vi "R2_Control.vi"() -> ()   [LabVIEW 2016]
uses:
  R2 Reactor Status v1.ctl
  R2 SBR Mode Control.ctl
  R2 pH Manual Control.ctl
  R2 Pump Manual Control.ctl
  R2 DO Manual Control.ctl
  R2Variables.lvlib
panel:
  in  "High DO Manual Control":cluster{"Air Valve":bool, "N2 Valve":bool}
  in  "High DO Control":T1={"DO set point (mg/L)"=2.0, "N2 Gain"=15.0, "Air Gain"=3.0, "DO Tolerance (mg/L)"=0.05, "Air Short Reaction Time (s)"=15.0, "Long Reaction Time (s)"=30.0, "N2 Short Reaction Time (s) 2"=10.0}
  out "Elapsed Time":dbl
  in  "Main DO Control":T1={"DO set point (mg/L)"=2.0, "N2 Gain"=15.0, "Air Gain"=5.0, "DO Tolerance (mg/L)"=0.05, "Air Short Reaction Time (s)"=15.0, "Long Reaction Time (s)"=30.0, "N2 Short Reaction Time (s) 2"=10.0}
  out "pH and DO":cluster{"pH":dbl, "DO (mg/L)":dbl}(graph)
  out "DO Intercept":dbl
  out "DO Slope":dbl
  out "pH Intercept":dbl
  out "pH Slope":dbl
  in  "DO Control":T2
  in  "Reactor 2 Pumps Manual Control":T3
  in  "pH Control":T4
  in  "pH Control":T5={" pH Set Point"=7.5, " pH Tolerance"=0.1, "Reaction Time (s)"=15.0, "Pump On Time (s)"=3.0}
  in  "SBR Timing":T6={"Anaerobic Feed"=60.0, "Aerobic"=180.0, "Settle 1"=3.0, "Floc Decant 1"=1.0, "Mix 2"=1.0, "Idle"=13.0, "Aerobic no DO control "=2.0, "Settle 2 (min)"=2.0, "Floc Decant 2"=1.0, "Mix 3"=1.0, "Settle 3"=1.0, "Floc Decant 3"=1.0, "Water Fill + Floc Return"=2.0, "High DO"=60.0, "N2 Purge"=5.0, "Effluent"=2.0}
  out "N2 and Air Flow":cluster{"N2 Flow":dbl, "Air Flow":dbl}(graph)
  out "Reactor 2 Status":T7 {"Compressed Air" format="%#.0g"; "Release Flow" format="%#.0g"; "DO Amp (A)" format="%#.4g"; "pH Amp (A)" format="%#.4g"; "DO (mg/L)" format="%#.2g"; "pH" format="%#.2g"}
  in  "Pumps Manual Control":bool
  in  "DO Manual Control":bool
  in  "pH Manual Control":bool
  in  "DO Calibrate":bool
  in  "pH Calibrate":bool
  # "On: Manual Mode\nOff: SBR Mode"
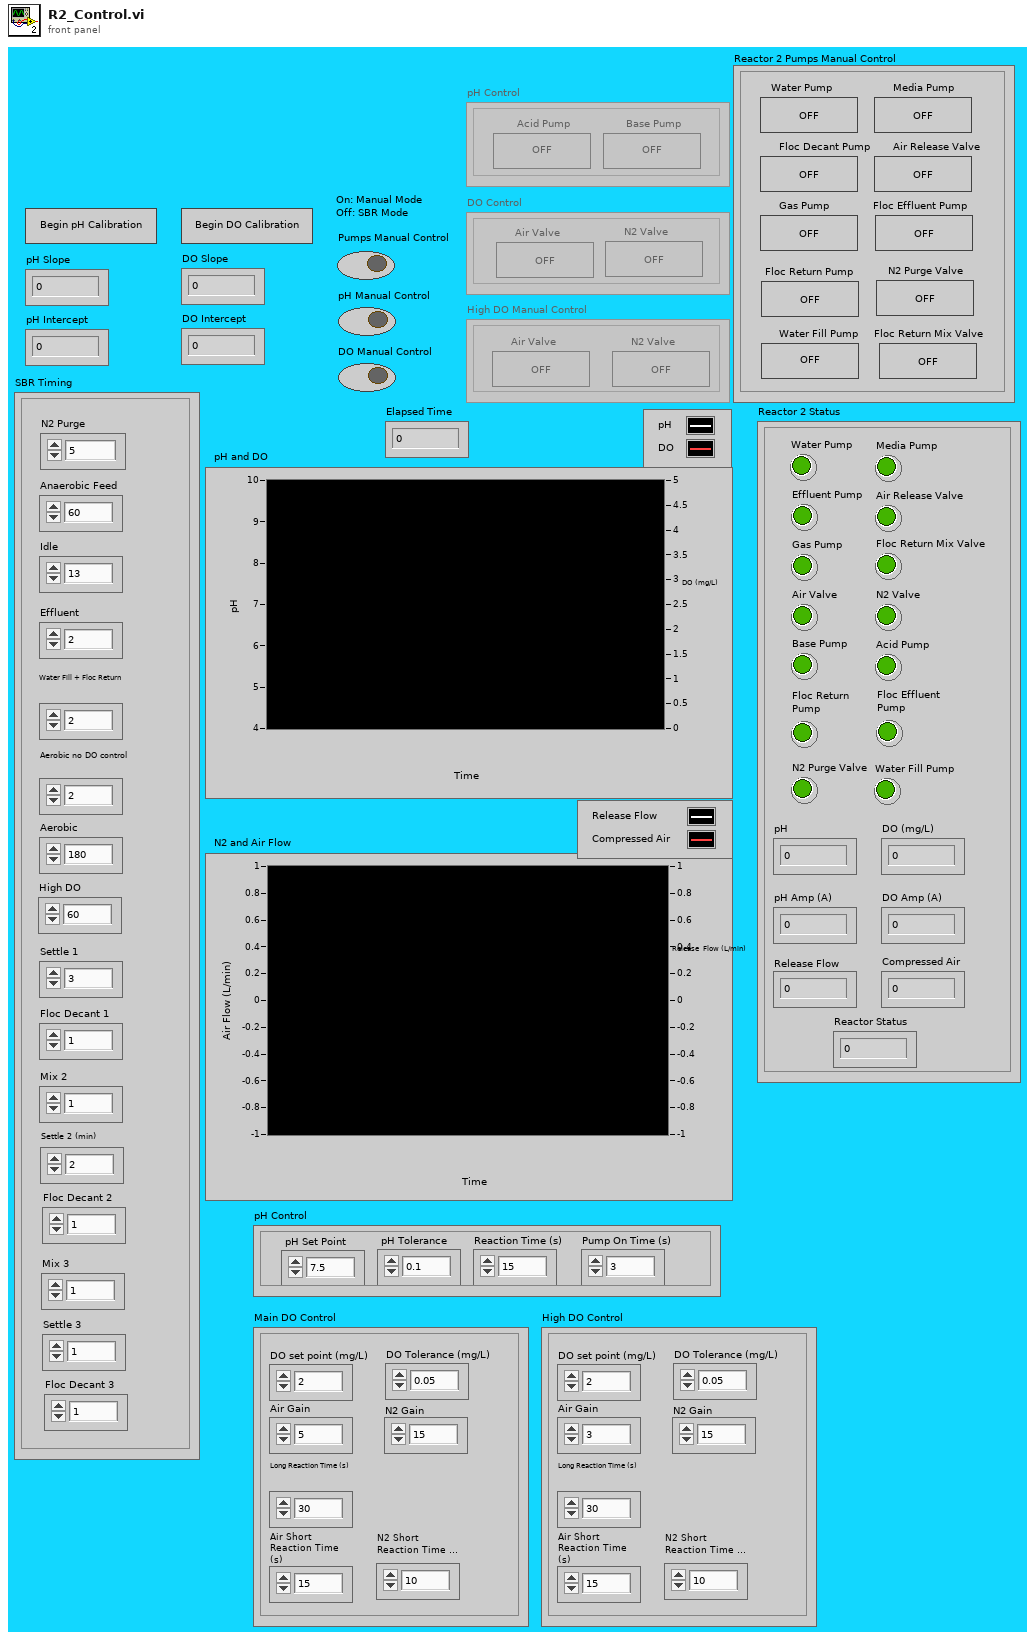
[diagram p1: front panel]
types:
  T1 = cluster{"DO set point (mg/L)":dbl, "N2 Gain":dbl, "Air Gain":dbl, "DO Tolerance (mg/L)":dbl, "Air Short Reaction Time (s)":dbl, "Long Reaction Time (s)":dbl, "N2 Short Reaction Time (s) 2":dbl}
  T2 = typedef "R2Variables.lvlib/R2 DO Manual Control.ctl" = cluster{"Air Valve":bool, "N2 Valve":bool}
  T3 = typedef "R2Variables.lvlib/R2 Pump Manual Control.ctl" = cluster{"Water Fill Pump":bool, "Floc Decant Pump":bool, "Media Pump":bool, "Gas Pump":bool, "Air Release Valve":bool, "Floc Effluent Pump":bool, "Floc Return Pump":bool, "N2 Purge Valve":bool, "Water Pump":bool, "Floc Return Mix Valve":bool}
  T4 = typedef "R2Variables.lvlib/R2 pH Manual Control.ctl" = cluster{"Acid Pump":bool, "Base Pump":bool}
  T5 = cluster{" pH Set Point":dbl, " pH Tolerance":dbl, "Reaction Time (s)":dbl, "Pump On Time (s)":dbl}
  T6 = typedef "R2Variables.lvlib/R2 SBR Mode Control.ctl" = cluster{"Anaerobic Feed":dbl, "Aerobic":dbl, "Settle 1":dbl, "Floc Decant 1":dbl, "Mix 2":dbl, "Idle":dbl, "Aerobic no DO control ":dbl, "Settle 2 (min)":dbl, "Floc Decant 2":dbl, "Mix 3":dbl, "Settle 3":dbl, "Floc Decant 3":dbl, "Water Fill + Floc Return":dbl, "High DO":dbl, "N2 Purge":dbl, "Effluent":dbl}
  T7 = typedef "R2Variables.lvlib/R2 Reactor Status v1.ctl" = cluster{"Water Fill Pump":bool, "Media Pump":bool, "Effluent Pump":bool, "Base Pump":bool, "Gas Pump":bool, "Acid Pump":bool, "Air Release Valve":bool, "N2 Valve":bool, "pH":dbl, "DO (mg/L)":dbl, "pH Amp (A)":dbl, "DO Amp (A)":dbl, "Release Flow":dbl, "Compressed Air":dbl, "Reactor Status":sgl, "Air Valve":bool, "Floc Return \nPump":bool, "Floc Effluent\nPump ":bool, "N2 Purge Valve":bool, "Water Pump":bool, "Floc Return Mix Valve":bool}
  T8 = enum8{"Enabled", "Disabled", "Disabled and Grayed Out"}
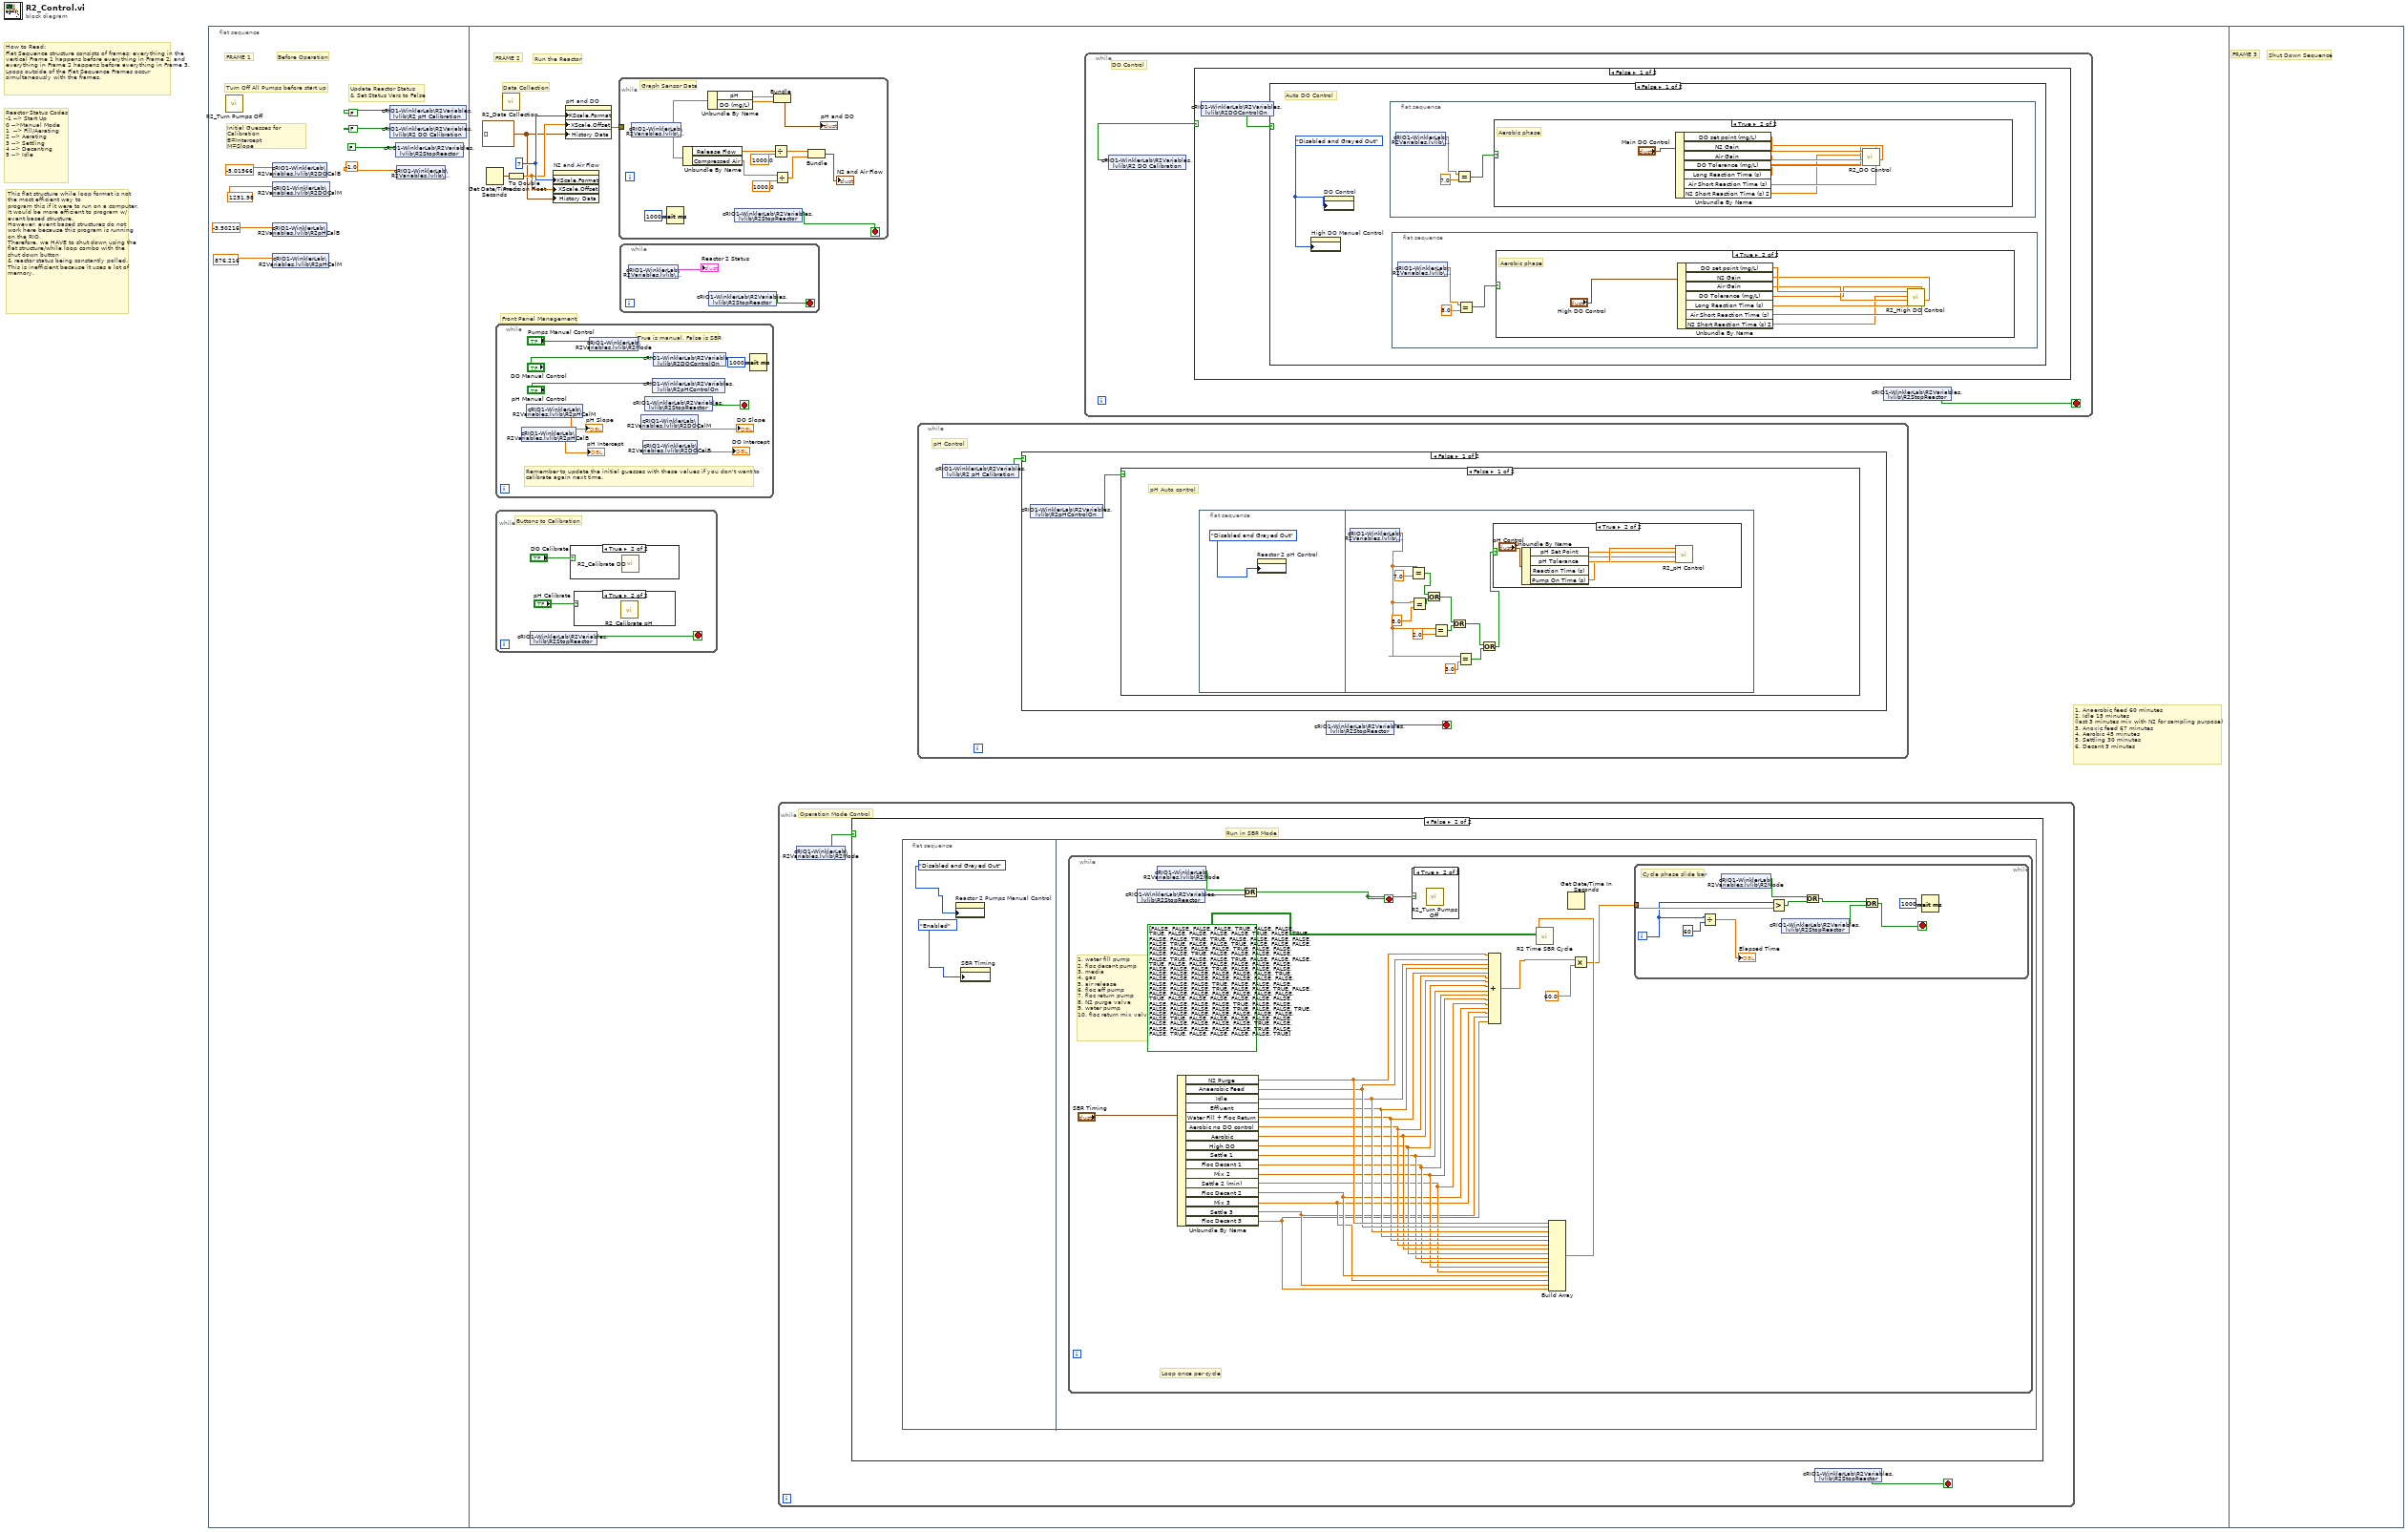
[diagram p0: block diagram]
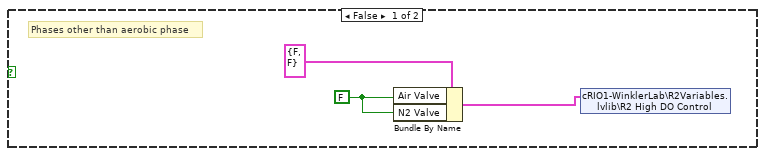
[diagram p2: hidden frame]
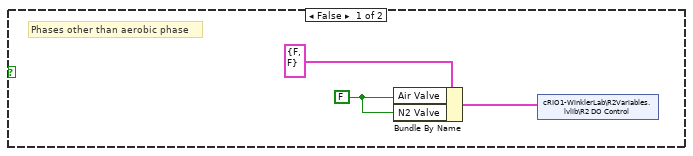
[diagram p3: hidden frame]
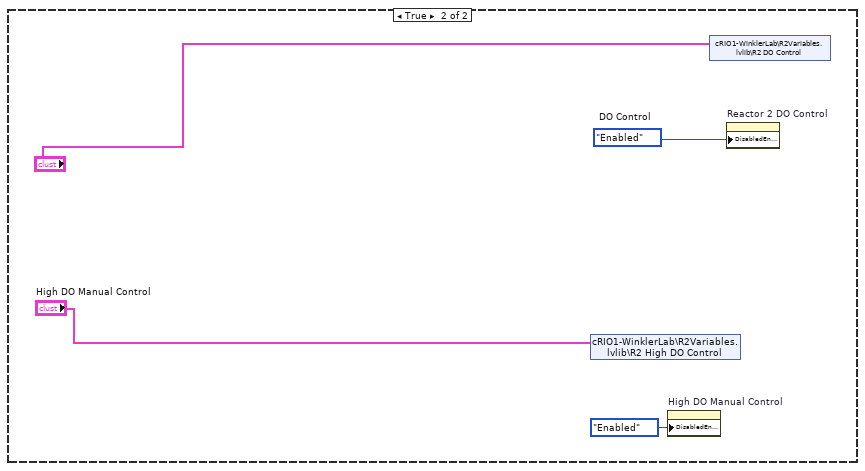
[diagram p4: hidden frame]
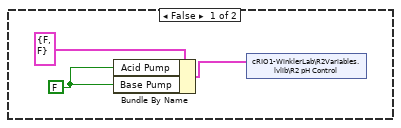
[diagram p8: hidden frame]
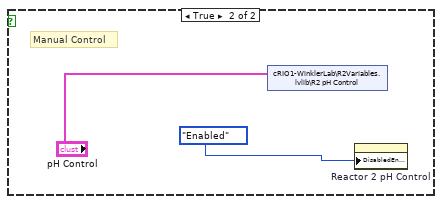
[diagram p9: hidden frame]
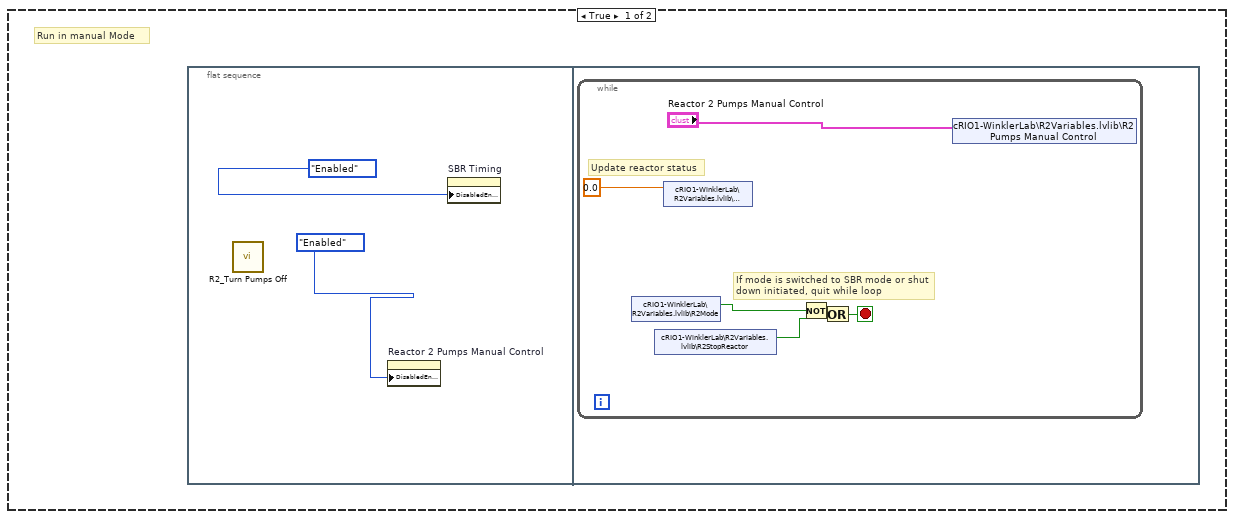
[diagram p11: hidden frame]
diagram:
  # "Reactor Status Codes\n-1 --> Start Up\n0 -->Manual Mode\n1  --> Fill/Aerating\n2 --> Aerating\n3 --> Settling\n4 --> Decanting\n5 --> Idle"
  # "How to Read:\nFlat Sequence structure consists of frames; everything in the vertical Frame 1 happens before everything in Frame 2, and everything in Frame 2 happens before everything in Frame 3.\nLoops outside of the Flat Sequence Frames occur simultaneously with the frames."
  # "This flat structure while loop format is not the most efficient way to \nprogram this if it were to run on a computer.\nIt would be more efficient to program w/ event based structure.\nHowever, event based structures do not work here because this program is running on the RIO.\nTherefore, we HAVE to shut down using the flat structure/while loop combo with the shut down button \n& reactor status being constantly polled.\nThis is inefficient because it uses a lot of memory."
  n1 = flat-sequence {
    frame #0 {
      # "Initial Guesses for Calibration\nB=Intercept\nM=Slope"
      # "Update Reactor Status \n& Set Status Vars to False"
      # "Turn Off All Pumps before start up"
      # "FRAME 1"
      # "Before Operation"
      n2 = call "R2_Turn Pumps Off.vi"() -> ()  [unwired: 12 in]
      n3 = shared-variable "cRIO1-WinklerLab\\R2Variables.lvlib\\R2DOCalB"(-5.01566 ("R1DOxCalB")) -> ()  [unwired: 1 in, 1 out]
      n4 = shared-variable "cRIO1-WinklerLab\\R2Variables.lvlib\\R2DOCalM"(1251.98 ("R1DOxCalM")) -> ()  [unwired: 1 in, 1 out]
      n5 = shared-variable "cRIO1-WinklerLab\\R2Variables.lvlib\\R2pHCalB"(-3.50216 ("R1pHCalB")) -> ()  [unwired: 1 in, 1 out]
      n6 = shared-variable "cRIO1-WinklerLab\\R2Variables.lvlib\\R2pHCalM"(876.216 ("R1pHCalM")) -> ()  [unwired: 1 in, 1 out]
      n7 = shared-variable "cRIO1-WinklerLab\\R2Variables.lvlib\\R2 pH Calibration"(FALSE ("pH Calibration")) -> ()  [unwired: 1 in, 1 out]
      n8 = shared-variable "cRIO1-WinklerLab\\R2Variables.lvlib\\R2 DO Calibration"(FALSE ("DO Calibration")) -> ()  [unwired: 1 in, 1 out]
      n9 = shared-variable "cRIO1-WinklerLab\\R2Variables.lvlib\\R2StopReactor"(FALSE ("R1Stop Reactor")) -> ()  [unwired: 1 in, 1 out]
      n10 = shared-variable "cRIO1-WinklerLab\\R2Variables.lvlib\\R2Phase"(-1.0) -> ()  [unwired: 1 in, 1 out]
    }
    frame #1 {
      w9 = cluster{"pH":dbl, "DO (mg/L)":dbl}[] [] ("History Data")
      w11 = u8 7 ("X Scale.Display Format:Format")
      # "1. Anaerobic feed 60 minutes\n2. Idle 15 minutes \n(last 3 minutes mix with N2 for sampling purpose)\n3. Anoxic feed 67 minutes\n4. Aerobic 45 minutes\n5. Settling 30 minutes\n6. Decant 5 minutes"
      # "Front Panel Management"
      # "Data Collection"
      # "FRAME 2"
      # "Run the Reactor"
      n11 = Get Date/Time In Seconds() -> (seconds since 1Jan1904=w13:timestamp)
      n12 = while {
        stop <- w98 stop-if-true
        # "Remember to update the initial guesses with these values if you don't want to calibrate again next time."
        # "True is manual, False is SBR"
        n13 = shared-variable "cRIO1-WinklerLab\\R2Variables.lvlib\\R2pHCalB"() -> (→"pH Intercept":dbl)  [unwired: 1 in, 1 out]
        n14 = shared-variable "cRIO1-WinklerLab\\R2Variables.lvlib\\R2pHCalM"() -> (→"pH Slope":dbl)  [unwired: 1 in, 1 out]
        n15 = shared-variable "cRIO1-WinklerLab\\R2Variables.lvlib\\R2Mode"("Pumps Manual Control") -> ()  [unwired: 1 in, 1 out]
        n16 = shared-variable "cRIO1-WinklerLab\\R2Variables.lvlib\\R2DOCalM"() -> (→"DO Slope":dbl)  [unwired: 1 in, 1 out]
        n17 = shared-variable "cRIO1-WinklerLab\\R2Variables.lvlib\\R2DOCalB"() -> (→"DO Intercept":dbl)  [unwired: 1 in, 1 out]
        n18 = shared-variable "cRIO1-WinklerLab\\R2Variables.lvlib\\R2StopReactor"() -> (w98:bool)  [unwired: 1 in, 1 out]
        n19 = shared-variable "cRIO1-WinklerLab\\R2Variables.lvlib\\R2pHControlOn"("pH Manual Control") -> ()  [unwired: 1 in, 1 out]
        n20 = shared-variable "cRIO1-WinklerLab\\R2Variables.lvlib\\R2DOControlOn"("DO Manual Control") -> ()  [unwired: 1 in, 1 out]
        n21 = Wait (ms)(milliseconds to wait=u32 1000) -> ()  [unwired: 1 out]
      }
      n22 = while {
        stop <- w65 stop-if-true
        # "Buttons to Calibration"
        n23 = shared-variable "cRIO1-WinklerLab\\R2Variables.lvlib\\R2StopReactor"() -> (w65:bool)  [unwired: 1 in, 1 out]
        n24 = case shown="True" "DO Calibrate" {
          frame False {
          }
          frame True {
            n25 = call "R2_Calibrate DO.vi"() -> ()  [unwired: 12 in]
          }
        }
        n26 = case shown="True" "pH Calibrate" {
          frame False {
          }
          frame True {
            n27 = call "R2_Calibrate pH.vi"() -> ()  [unwired: 12 in]
          }
        }
      }
      n28 = call "R2_Data Collection.vi"() -> ()  [unwired: 12 in]
      n29 = To Double Precision Float(number=w13) -> (double precision float=w10:dbl)
      n30 = property on="N2 and Air Flow" class="WFChart (strict)"("XScale.Format"=w11, "XScale.Offset"=w10, "History Data"=w9) -> ()  [unwired: 2 in, 2 out]
      n31 = property on="pH and DO" class="WFChart (strict)"("XScale.Format"=w11, "XScale.Offset"=w10, "History Data"=w9) -> (error out=w12:errorcluster)  [unwired: 2 in, 1 out]
      n32 = while {
        tunnel: w12 -> [_]
        stop <- w24 stop-if-true
        # "Graph Sensor Data"
        n33 = shared-variable "cRIO1-WinklerLab\\R2Variables.lvlib\\R2Status"() -> (w25:T7)  [unwired: 1 in, 1 out]
        n34 = Wait (ms)(milliseconds to wait=u32 1000) -> ()  [unwired: 1 out]
        n35 = Unbundle By Name(w25) -> ("Release Flow"=w21:dbl, "Compressed Air"=w18:dbl)
        n36 = Unbundle By Name(w25) -> ("pH"=w26:dbl, "DO (mg/L)"=w27:dbl)
        n37 = shared-variable "cRIO1-WinklerLab\\R2Variables.lvlib\\R2StopReactor"() -> (w24:bool)  [unwired: 1 in, 1 out]
        n38 = Divide(x=w21, y=1000.0) -> (x/y=w17:dbl)
        n39 = Bundle("pH"=w26, "DO (mg/L)"=w27) -> (→"pH and DO":cluster{"pH":dbl, "DO (mg/L)":dbl})  [unwired: 1 in]
        n40 = Divide(x=w18, y=1000.0) -> (x/y=w16:dbl)
        n41 = Bundle(w17, w16) -> (→"N2 and Air Flow":cluster{dbl, dbl})  [unwired: 1 in]
      }
      n42 = while {
        stop <- w14 stop-if-true
        n43 = shared-variable "cRIO1-WinklerLab\\R2Variables.lvlib\\R2Status"() -> (→"Reactor 2 Status":T7)  [unwired: 1 in, 1 out]
        n44 = shared-variable "cRIO1-WinklerLab\\R2Variables.lvlib\\R2StopReactor"() -> (w14:bool)  [unwired: 1 in, 1 out]
      }
      n45 = while {
        stop <- w104 stop-if-true
        # "Operation Mode Control"
        n46 = shared-variable "cRIO1-WinklerLab\\R2Variables.lvlib\\R2Mode"() -> (w103:bool)  [unwired: 1 in, 1 out]
        n47 = case shown="False" w103 {
          frame True {
            # "Run in manual Mode"
            n48 = flat-sequence {
              frame #0 {
                n49 = call "R2_Turn Pumps Off.vi"() -> ()  [unwired: 12 in]
                n50 = property on="Reactor 2 Pumps Manual Control" class="Clust (strict)"("DisabledEnum"=T8."Enabled" ("Disabled")) -> ()  [unwired: 2 in, 2 out]
                n51 = property on="SBR Timing" class="Clust (strict)"("DisabledEnum"=T8."Enabled" ("Disabled")) -> ()  [unwired: 2 in, 2 out]
              }
              frame #1 {
                n52 = while {
                  stop <- w111 stop-if-true
                  # "If mode is switched to SBR mode or shut \ndown initiated, quit while loop"
                  # "Update reactor status"
                  n53 = shared-variable "cRIO1-WinklerLab\\R2Variables.lvlib\\R2Mode"() -> (w109:bool)  [unwired: 1 in, 1 out]
                  n54 = shared-variable "cRIO1-WinklerLab\\R2Variables.lvlib\\R2StopReactor"() -> (w108:bool)  [unwired: 1 in, 1 out]
                  n55 = shared-variable "cRIO1-WinklerLab\\R2Variables.lvlib\\R2Phase"(0.0 ("Reactor Status")) -> ()  [unwired: 1 in, 1 out]
                  n56 = Not(x=w109) -> (.not. x?=w112:bool)
                  n57 = Or(x=w112, y=w108) -> (x .or. y?=w111:bool)
                  n58 = shared-variable "cRIO1-WinklerLab\\R2Variables.lvlib\\R2 Pumps Manual Control"("Reactor 2 Pumps Manual Control") -> ()  [unwired: 1 in, 1 out]
                }
              }
            }
          }
          frame False {
            # "Run in SBR Mode"
            n59 = flat-sequence {
              frame #0 {
                n60 = property on="Reactor 2 Pumps Manual Control" class="Clust (strict)"("DisabledEnum"=T8."Disabled and Grayed Out" ("Disabled")) -> ()  [unwired: 2 in, 2 out]
                n61 = property on="SBR Timing" class="Clust (strict)"("DisabledEnum"=T8."Enabled" ("Disabled")) -> ()  [unwired: 2 in, 2 out]
              }
              frame #1 {
                n62 = while {
                  stop <- w139 stop-if-true
                  # "1. water fill pump \n2. floc decant pump\n3. media \n4. gas \n5. air release\n6. floc eff pump\n7. floc return pump\n8. N2 purge valve\n9. water pump\n10. floc return mix valve"
                  # "Loop once per cycle"
                  n63 = shared-variable "cRIO1-WinklerLab\\R2Variables.lvlib\\R2StopReactor"() -> (w137:bool)  [unwired: 1 in, 1 out]
                  n64 = shared-variable "cRIO1-WinklerLab\\R2Variables.lvlib\\R2Mode"() -> (w138:bool)  [unwired: 1 in, 1 out]
                  n65 = Unbundle By Name("SBR Timing") -> ("N2 Purge"=w130:dbl, "Anaerobic Feed"=w129:dbl, "Idle"=w128:dbl, "Effluent"=w127:dbl, "Water Fill + Floc Return"=w126:dbl, "Aerobic no DO control"=w125:dbl, "Aerobic"=w124:dbl, "High DO"=w123:dbl, "Settle 1"=w122:dbl, "Floc Decant 1"=w121:dbl, "Mix 2"=w120:dbl, "Settle 2 (min)"=w119:dbl, "Floc Decant 2"=w118:dbl, "Mix 3"=w117:dbl, "Settle 3"=w116:dbl, "Floc Decant 3"=w115:dbl)
                  n66 = Or(x=w138, y=w137) -> (x .or. y?=w139:bool)
                  n67 = case shown="True" w139 {
                    frame False {
                    }
                    frame True {
                      n68 = call "R2_Turn Pumps Off.vi"() -> ()  [unwired: 12 in]
                    }
                  }
                  n69 = Compound Arithmetic op=ADD(w130, w129, w128, w127, w126, w125, w124, w123, w122, w121, w120, w119, w118, w117, w116, w115) -> (w132:dbl)
                  n70 = Build Array(w130, w129, w128, w127, w126, w125, w124, w123, w122, w121, w120, w119, w118, w117, w116, w115) -> (w135:dbl[])
                  n71 = call "R2 Time SBR Cycle.vi"("Pump Status Array"=bool[][] [[FALSE, FALSE, FALSE, FALSE, TRUE, FALSE, FALSE, TRUE, FALSE, FALSE], [FALSE, FALSE, TRUE, FALSE, TRUE, FALSE, FALSE, TRUE, TRUE, FALSE], [FALSE, FALSE, FALSE, FALSE, TRUE, FALSE, FALSE, TRUE, FALSE, FALSE], [FALSE, FALSE, FALSE, FALSE, FALSE, TRUE, FALSE, FALSE, FALSE, FALSE], [TRUE, FALSE, FALSE, FALSE, FALSE, FALSE, TRUE, FALSE, FALSE, TRUE], [FALSE, FALSE, FALSE, TRUE, FALSE, FALSE, FALSE, FALSE, FALSE, FALSE], [FALSE, FALSE, FALSE, TRUE, FALSE, FALSE, FALSE, FALSE, FALSE, FALSE], [FALSE, FALSE, FALSE, TRUE, FALSE, FALSE, FALSE, FALSE, FALSE, FALSE], [FALSE, FALSE, FALSE, FALSE, TRUE, FALSE, FALSE, FALSE, FALSE, FALSE], [FALSE, TRUE, FALSE, FALSE, TRUE, FALSE, FALSE, FALSE, FALSE, FALSE], [FALSE, FALSE, FALSE, TRUE, FALSE, FALSE, FALSE, FALSE, FALSE, FALSE], [FALSE, FALSE, FALSE, FALSE, TRUE, FALSE, FALSE, FALSE, FALSE, FALSE], [FALSE, TRUE, FALSE, FALSE, TRUE, FALSE, FALSE, FALSE, FALSE, FALSE], [FALSE, FALSE, FALSE, TRUE, FALSE, FALSE, FALSE, FALSE, FALSE, FALSE], [FALSE, FALSE, FALSE, FALSE, TRUE, FALSE, FALSE, FALSE, FALSE, FALSE], [FALSE, TRUE, FALSE, FALSE, TRUE, FALSE, FALSE, FALSE, FALSE, TRUE]], "Array"=w135) -> ()  [unwired: 10 in]
                  n72 = Get Date/Time In Seconds() -> ()  [unwired: 1 out]
                  n73 = Multiply(x=w132, y=60.0) -> (x*y=w133:dbl)
                  n74 = while {
                    tunnel: w133 -> [w148]
                    i -> [w141]
                    stop <- w142 stop-if-true
                    # "Cycle phase slide bar"
                    n75 = Divide(x=w141, y=60) -> (x/y=→"Elapsed Time":dbl)
                    n76 = shared-variable "cRIO1-WinklerLab\\R2Variables.lvlib\\R2Mode"() -> (w145:bool)  [unwired: 1 in, 1 out]
                    n77 = Greater?(x=w141, y=w148) -> (0:w146:bool)
                    n78 = shared-variable "cRIO1-WinklerLab\\R2Variables.lvlib\\R2StopReactor"() -> (w143:bool)  [unwired: 1 in, 1 out]
                    n79 = Or(x=w145, y=w146) -> (x .or. y?=w144:bool)
                    n80 = Or(x=w144, y=w143) -> (x .or. y?=w142:bool)
                    n81 = Wait (ms)(milliseconds to wait=u32 1000) -> ()  [unwired: 1 out]
                  }
                }
              }
            }
          }
        }
        n82 = shared-variable "cRIO1-WinklerLab\\R2Variables.lvlib\\R2StopReactor"() -> (w104:bool)  [unwired: 1 in, 1 out]
      }
      n83 = while {
        stop <- w69 stop-if-true
        # "pH Control"
        n84 = shared-variable "cRIO1-WinklerLab\\R2Variables.lvlib\\R2 pH Calibration"() -> (w68:bool)  [unwired: 1 in, 1 out]
        n85 = case shown="False" w68 {
          frame False {
            n86 = shared-variable "cRIO1-WinklerLab\\R2Variables.lvlib\\R2pHControlOn"() -> (w70:bool)  [unwired: 1 in, 1 out]
            n87 = case shown="False" w70 {
              frame False {
                # "pH Auto control"
                n88 = flat-sequence {
                  frame #0 {
                    n89 = property on="Reactor 2 pH Control" class="Clust (strict)"("DisabledEnum"=T8."Disabled and Grayed Out" ("Disabled")) -> ()  [unwired: 2 in, 2 out]
                  }
                  frame #1 {
                    n90 = shared-variable "cRIO1-WinklerLab\\R2Variables.lvlib\\R2Phase"() -> (w75:dbl)  [unwired: 1 in, 1 out]
                    n91 = Equal?(x=w75, y=7.0) -> (x = y?=w82:bool)
                    n92 = Equal?(x=w75, y=8.0) -> (x = y?=w81:bool)
                    n93 = Or(x=w82, y=w81) -> (x .or. y?=w79:bool)
                    n94 = Equal?(x=w75, y=2.0) -> (x = y?=w78:bool)
                    n95 = Or(x=w79, y=w78) -> (x .or. y?=w76:bool)
                    n96 = Equal?(x=w75, y=3.0) -> (x = y?=w74:bool)
                    n97 = Or(x=w76, y=w74) -> (x .or. y?=w73:bool)
                    n98 = case shown="True" w73 {
                      frame False {
                        w85 = FALSE
                        n99 = Bundle By Name(cluster=T4 {"Acid Pump"=FALSE, "Base Pump"=FALSE} ("Reactor 2 pH Control"), "Acid Pump"=w85, "Base Pump"=w85) -> (w84:T4)
                        n100 = shared-variable "cRIO1-WinklerLab\\R2Variables.lvlib\\R2 pH Control"(w84) -> ()  [unwired: 1 in, 1 out]
                      }
                      frame True {
                        n101 = Unbundle By Name("pH Control") -> ("pH Set Point"=w89:dbl, "pH Tolerance"=w90:dbl, "Reaction Time (s)"=w88:dbl, "Pump On Time (s)"=w87:dbl)
                        n102 = call "R2_pH Control.vi"("Pump On Time (s)"=w87, "Reaction Time (s)"=w88, "pH Set Point"=w89, "pH Tolerance"=w90) -> ()  [unwired: 8 in]
                      }
                    }
                  }
                }
              }
              frame True {
                # "Manual Control"
                n103 = shared-variable "cRIO1-WinklerLab\\R2Variables.lvlib\\R2 pH Control"("pH Control") -> ()  [unwired: 1 in, 1 out]
                n104 = property on="Reactor 2 pH Control" class="Clust (strict)"("DisabledEnum"=T8."Enabled" ("Disabled")) -> ()  [unwired: 2 in, 2 out]
              }
            }
          }
          frame True {
          }
        }
        n105 = shared-variable "cRIO1-WinklerLab\\R2Variables.lvlib\\R2StopReactor"() -> (w69:bool)  [unwired: 1 in, 1 out]
      }
      n106 = while {
        stop <- w30 stop-if-true
        # "DO Control"
        n107 = shared-variable "cRIO1-WinklerLab\\R2Variables.lvlib\\R2 DO Calibration"() -> (w29:bool)  [unwired: 1 in, 1 out]
        n108 = case shown="False" w29 {
          frame False {
            n109 = shared-variable "cRIO1-WinklerLab\\R2Variables.lvlib\\R2DOControlOn"() -> (w31:bool)  [unwired: 1 in, 1 out]
            n110 = case shown="False" w31 {
              frame False {
                w32 = T8."Disabled and Grayed Out" ("Disabled")
                # "Auto DO Control"
                n111 = property on="High DO Manual Control" class="Clust (strict)"("DisabledEnum"=w32) -> ()  [unwired: 2 in, 2 out]
                n112 = property on="DO Control" class="Clust (strict)"("DisabledEnum"=w32) -> ()  [unwired: 2 in, 2 out]
                n113 = flat-sequence {
                  frame #0 {
                    n114 = shared-variable "cRIO1-WinklerLab\\R2Variables.lvlib\\R2Phase"() -> (w49:dbl)  [unwired: 1 in, 1 out]
                    n115 = Equal?(x=w49, y=7.0) -> (x = y?=w47:bool)
                    n116 = case shown="True" w47 {
                      frame False {
                        w51 = FALSE
                        # "Phases other than aerobic phase"
                        n117 = Bundle By Name(cluster=T2 {"Air Valve"=FALSE, "N2 Valve"=FALSE} ("Reactor 2 DO Control"), "Air Valve"=w51, "N2 Valve"=w51) -> (w52:T2)
                        n118 = shared-variable "cRIO1-WinklerLab\\R2Variables.lvlib\\R2 DO Control"(w52) -> ()  [unwired: 1 in, 1 out]
                      }
                      frame True {
                        # "Aerobic phase"
                        n119 = Unbundle By Name("Main DO Control") -> ("DO set point (mg/L)"=w59:dbl, "N2 Gain"=w58:dbl, "Air Gain"=w57:dbl, "DO Tolerance (mg/L)"=w56:dbl, "Long Reaction Time (s)"=w55:dbl, "Air Short Reaction Time (s)"=w54:dbl, "N2 Short Reaction Time (s) 2"=w53:dbl)
                        n120 = call "R2_DO Control.vi"("Air Short Reaction Time (s)"=w54, "N2 Gain"=w58, "DO Tolerance (mg/L)"=w56, "Long Reaction Time (s)"=w55, "Air Gain"=w57, "N2 Short Reaction Time (s)"=w53, "DO Set Point (mg/L)"=w59) -> ()  [unwired: 1 in]
                      }
                    }
                  }
                }
                n121 = flat-sequence {
                  frame #0 {
                    n122 = shared-variable "cRIO1-WinklerLab\\R2Variables.lvlib\\R2Phase"() -> (w35:dbl)  [unwired: 1 in, 1 out]
                    n123 = Equal?(x=w35, y=8.0) -> (x = y?=w33:bool)
                    n124 = case shown="True" w33 {
                      frame False {
                        w38 = FALSE
                        # "Phases other than aerobic phase"
                        n125 = Bundle By Name(cluster=T2 {"Air Valve"=FALSE, "N2 Valve"=FALSE} ("Reactor 2 DO Control"), "Air Valve"=w38, "N2 Valve"=w38) -> (w36:T2)
                        n126 = shared-variable "cRIO1-WinklerLab\\R2Variables.lvlib\\R2 High DO Control"(w36) -> ()  [unwired: 1 in, 1 out]
                      }
                      frame True {
                        # "Aerobic phase"
                        n127 = Unbundle By Name("High DO Control") -> ("DO set point (mg/L)"=w45:dbl, "N2 Gain"=w44:dbl, "Air Gain"=w43:dbl, "DO Tolerance (mg/L)"=w42:dbl, "Long Reaction Time (s)"=w41:dbl, "Air Short Reaction Time (s)"=w40:dbl, "N2 Short Reaction Time (s) 2"=w39:dbl)
                        n128 = call "R2_High DO Control.vi"("Air Short Reaction Time (s)"=w40, "N2 Gain"=w44, "DO Tolerance (mg/L)"=w42, "Long Reaction Time (s)"=w41, "Air Gain"=w43, "N2 Short Reaction Time (s)"=w39, "DO Set Point (mg/L)"=w45) -> ()  [unwired: 1 in]
                      }
                    }
                  }
                }
              }
              frame True {
                n129 = shared-variable "cRIO1-WinklerLab\\R2Variables.lvlib\\R2 High DO Control"("High DO Manual Control") -> ()  [unwired: 1 in, 1 out]
                n130 = property on="High DO Manual Control" class="Clust (strict)"("DisabledEnum"=T8."Enabled" ("Disabled")) -> ()  [unwired: 2 in, 2 out]
                n131 = shared-variable "cRIO1-WinklerLab\\R2Variables.lvlib\\R2 DO Control"("DO Control") -> ()  [unwired: 1 in, 1 out]
                n132 = property on="Reactor 2 DO Control" class="Clust (strict)"("DisabledEnum"=T8."Enabled" ("Disabled")) -> ()  [unwired: 2 in, 2 out]
              }
            }
          }
          frame True {
          }
        }
        n133 = shared-variable "cRIO1-WinklerLab\\R2Variables.lvlib\\R2StopReactor"() -> (w30:bool)  [unwired: 1 in, 1 out]
      }
    }
    frame #2 {
      # "FRAME 3"
      # "Shut Down Sequence"
    }
  }
